vi "Process.vi"(0 "InteractionProcessor in":refnum<class "InteractionProcessor.lvclass">, 5 "Internal Message Queue":refnum<queue>, 7 "Wait Time":u32 caption="ms" step=1, 9 "Results Notifier":refnum<notifier>, 11 "error in (no error)":errorcluster) -> (4 "InteractionProcessor out":refnum<class "InteractionProcessor.lvclass">, 15 "error out":errorcluster)   [LabVIEW 2023, in "HAF.lvlib" / "InteractionProcessor.lvclass"]
doc: "Process all Command Directors. These are iterated through once and told to process the Commands they hold. Those Command Directors that are Done, are not processed but skipped over. Each pass results in a Continue Message being placed on the queue so the Main Processing Loop can continue."
uses:
  InteractionProcessor.lvclass
  ReadCommand/ReadCommand.lvclass
  Message.ctl
  All Internal Message Ids.ctl
  CommandDirector/CommandDirector.lvclass
  InteractionProcessor.lvclass/InteractionProcessor.ctl
  HAF.lvlib
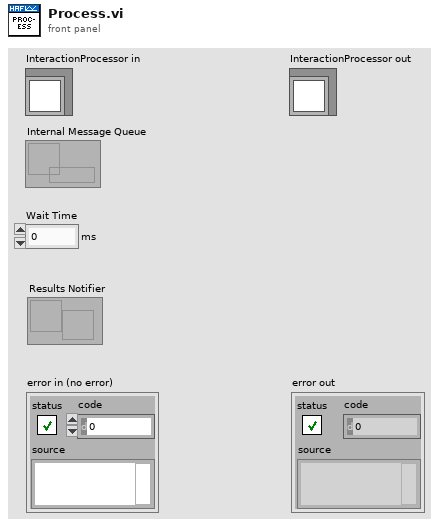
[diagram p1: front panel]
types:
  T1 = typedef "HAF.lvlib/All Internal Message Ids.ctl" = cluster{"Initialise":string, "Process":string, "Continue":string, "Done":string, "Pause":string, "Resume":string, "Stop":string, "Exit":string, "Inject":string}
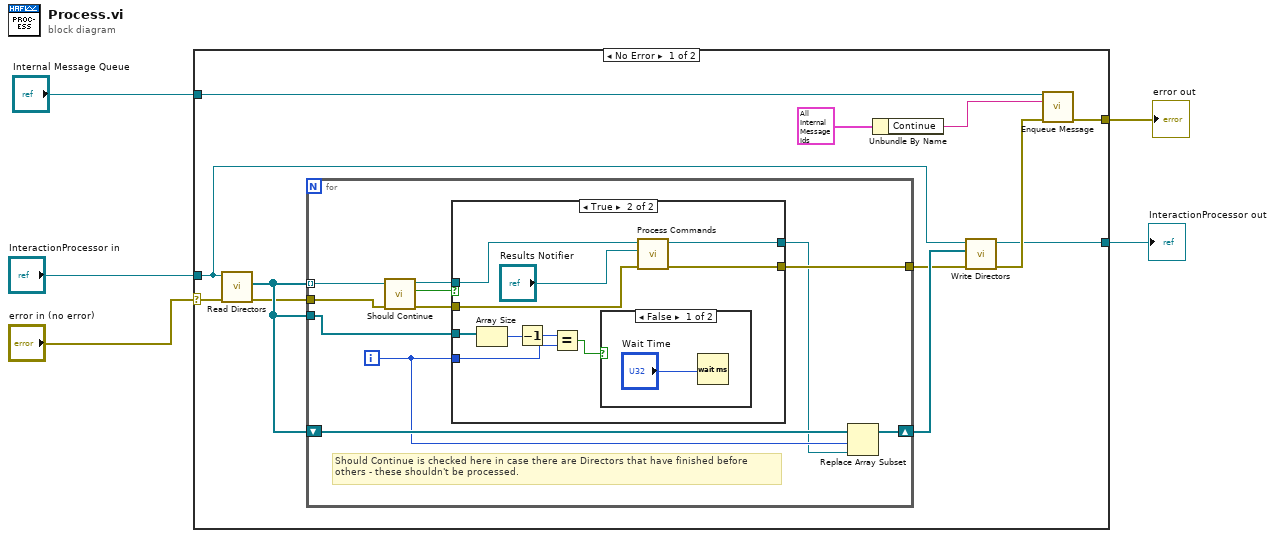
[diagram p0: block diagram]
diagram:
  n1 = case shown="No Error" "error in (no error)" {
    selector: "error in (no error)" -> [w17 w43]
    tunnel: [w9 w43] -> w1
    tunnel: "InteractionProcessor in" -> [w12 w42]
    tunnel: "Internal Message Queue" -> [w10 _]
    tunnel: [w8 w42] -> w2
    frame No Error {
      n2 = call-dynamic "Read Directors.vi"("error in (no error)"=w17, "InteractionProcessor in"=w12) -> ("error out"=w15:errorcluster, "Directors"=w16:refnum<class "CommandDirector.lvclass">[])  [unwired: 7 in, 1 out]
      n3 = for {
        tunnel: w16 -> [w28] mode=indexing
        tunnel: w16 -> [w23]
        shift-right: [w18] -> w14
        shift-left: w16 -> [w21]
        tunnel: w15 -> [w27]
        tunnel: [w22] -> w13
        i -> [w20]
        # "Should Continue is checked here in case there are Directors that have finished before\nothers - these shouldn't be processed."
        n4 = call-dynamic "Should Continue.vi"("error in (no error)"=w27, "CommandDirector in"=w28) -> ("error out"=w24:errorcluster, "Should Continue"=w26:bool, "CommandDirector out"=w25:refnum<class "CommandDirector.lvclass">)  [unwired: 7 in]
        n5 = case shown="True" w26 {
          tunnel: w25 -> [w29 w35]
          tunnel: w24 -> [w30 w34]
          tunnel: w23 -> [_ w40]
          tunnel: w20 -> [_ w37]
          tunnel: [w29 w32] -> w19
          tunnel: [w30 w31] -> w22
          frame False {
            # "This Director has Done so do nothing."
          }
          frame True {
            n6 = Array Size(array=w40) -> (size(s)=w39:i32)
            n7 = Decrement(x=w39) -> (x-1=w38:i32)
            n8 = Equal?(x=w38, y=w37) -> (x = y?=w36:bool)
            n9 = case shown="False" w36 {
              frame False {
                n10 = Wait (ms)(milliseconds to wait="Wait Time") -> ()  [unwired: 1 out]
              }
              frame True {
              }
            }
            n11 = call-dynamic "Process Commands.vi"("error in (no error)"=w34, "Results Notifier"="Results Notifier", "CommandDirector in"=w35) -> ("error out"=w31:errorcluster, "CommandDirector out"=w32:refnum<class "CommandDirector.lvclass">)  [unwired: 7 in]
          }
        }
        n12 = Replace Array Subset(array=w21, new element=w19, index=w20) -> (w18:refnum<class "CommandDirector.lvclass">[])
      }
      n13 = Unbundle By Name(T1 {"Initialise"="Initialise", "Process"="Process", "Continue"="Continue", "Done"="Done", "Pause"="Pause", "Resume"="Resume", "Stop"="Stop", "Exit"="Exit", "Inject"=""} ("Message Ids")) -> ("Continue"=w6:string)
      n14 = call-dynamic "Write Directors.vi"("error in (no error)"=w13, "Directors"=w14, "InteractionProcessor in"=w12) -> ("error out"=w11:errorcluster, "InteractionProcessor out"=w8:refnum<class "InteractionProcessor.lvclass">)  [unwired: 7 in]
      n15 = call "Enqueue Message.vi"("Message Queue In"=w10, "Message Id"=w6, "error in (no error)"=w11) -> ("error out"=w9:errorcluster)  [unwired: 11 in, 1 out]
    }
    frame Error {
    }
  }
  "error out" <- w1
  "InteractionProcessor out" <- w2
